vi "Untitled 1.vi"() -> ()   [LabVIEW 2015]
uses:
  <instrlib>/Fluke 289/Fluke 289.lvlib
panel:
  in  "stop":bool
  out "Attribute":string
  out "State":string
  out "Unit":string
  out "Reading Value":dbl
  in  "VISA resource name":refnum<visa-resource-name>
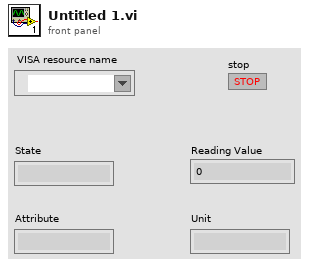
[diagram p1: front panel]
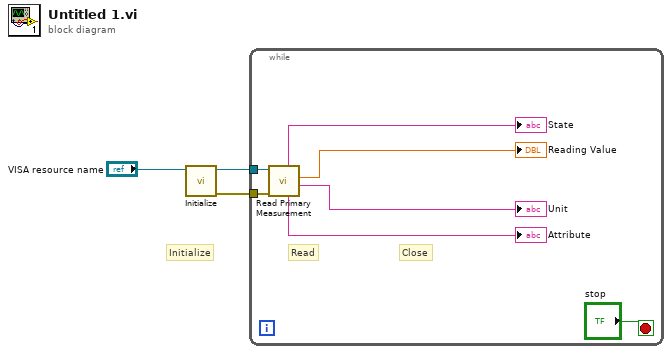
[diagram p0: block diagram]
diagram:
  # "Initialize"
  n1 = call <instrlib>:"Initialize.vi"("VISA resource name"="VISA resource name") -> ("error out"=w1:errorcluster, "VISA resource name out"=w2:refnum<visa-resource-name>)  [unwired: 9 in]
  n2 = while {
    tunnel: w2 -> [w10]
    tunnel: w1 -> [w9]
    stop <- "stop" stop-if-true
    # "Read"
    # "Close"
    n3 = call <instrlib>:"Read Primary Measurement.vi"("error in (no error)"=w9, "VISA resource name"=w10) -> ("Unit"=→"Unit":string, "Reading Value"=→"Reading Value":dbl, "Attribute"=→"Attribute":string, "State"=→"State":string)  [unwired: 4 in, 2 out]
  }
